vi "Create a constant from terminal.vi"(5 "Terminal Sink":refnum<vi>, 8 "error in (no error)":errorcluster, 10 "Value":variant, 11 "Constant from this terminal":refnum<vi>) -> (0 "error out":errorcluster, 2 "Terminal":refnum<vi>, 3 "Const Refnum":refnum<vi>)   [LabVIEW 2014, in "Scripting Tools.lvlib"]
doc: "Create a constant based on the type of <b>Constant from this terminal</b>. If <b>Value</b> is wired with the same type as the terminal, then the constant has the name and value of this data rather than the name and value associated with the terminal."
uses:
  <userlib>/_LAVACR/Scripting Tools/Scripting Tools.lvlib
  <vilib>/Utility/VariantDataType/VariantType.lvlib
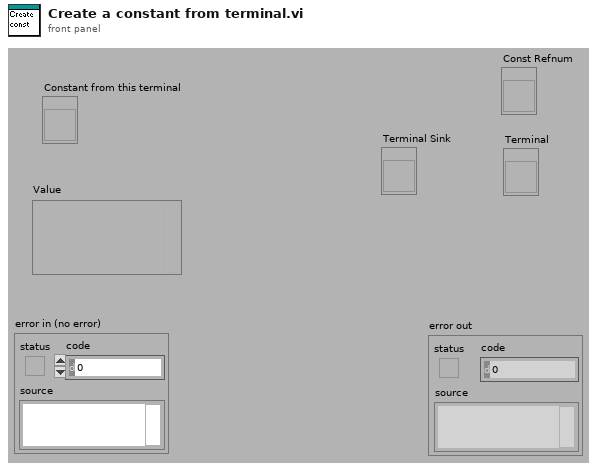
[diagram p1: front panel]
types:
  T1 = typedef "VariantType.lvlib/Type.ctl" = enum8{"Invalid Type", "Void", "I8", "I16", "I32", "I64", "U8", "U16", "U32", "U64", "Single Float", "Double Float", "Extended Float", "Single Complex", "Double Complex", "Extended Complex", "Enum U8", "Enum U16", "Enum U32", "Enum U64", "Single Float With Unit", "Double Float With Unit", "Extended Float With Unit", "Single Complex with Unit", "Double Complex with Unit", "Extended Complex with Unit", "Boolean", "String", "Path", "Picture", "Tag", "Array", "Cluster", "Variant", "LV Variant", "Waveform", "Timestamp", "Digital Waveform", "Digital Data", "ExpressData", "Refnum", "External Data", "VI", "Poly VI", "LabVIEW Class Instance", "Fixed Point"}
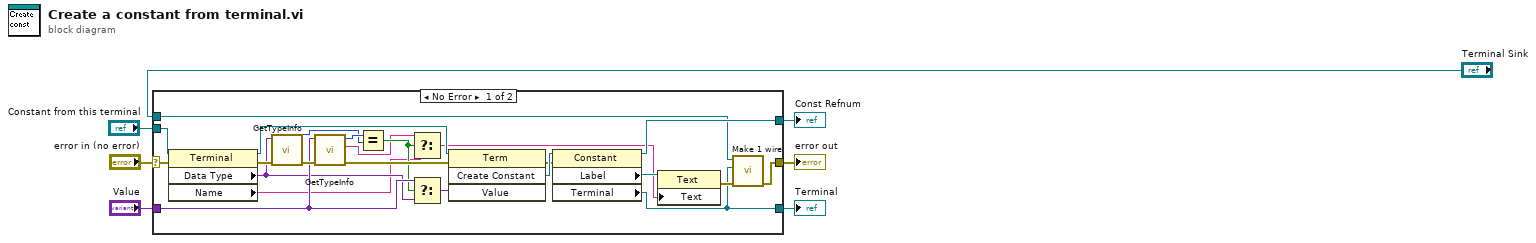
[diagram p0: block diagram]
diagram:
  n1 = case shown="No Error" "error in (no error)" {
    selector: "error in (no error)" -> [w18 w31]
    tunnel: [w29 w31] -> w6
    tunnel: [w27 _] -> w4
    tunnel: [w30 _] -> w5
    tunnel: "Terminal Sink" -> [w26 _]
    tunnel: "Constant from this terminal" -> [w19 _]
    tunnel: "Value" -> [w15 _]
    frame No Error {
      n2 = property class="Terminal"(reference=w19, error in=w18) -> (reference out=w20:refnum<vi>, error out=w22:errorcluster, "Data Type"=w14:variant, "Name"=w9:string)
      n3 = call <vilib>:"GetTypeInfo.vi"("error in (no error)"=w22, "Variant"=w14) -> ("error out"=w21:errorcluster, "Type Enum"=w16:T1)  [unwired: 8 out]
      n4 = call <vilib>:"GetTypeInfo.vi"("error in (no error)"=w21, "Variant"=w15) -> ("error out"=w12:errorcluster, "Name"=w10:string, "Type Enum"=w17:T1)  [unwired: 7 out]
      n5 = Equal?(x=w17, y=w16) -> (x = y?=w11:bool)
      n6 = Select(t=w10, s=w11, f=w9) -> (s? t:f=w8:string)
      n7 = Select(t=w15, s=w11, f=w14) -> (s? t:f=w13:variant)
      n8 = invoke class="Term" method="Create Constant"(reference=w20, error in=w12, "Value"=w13) -> (error out=w23:errorcluster, "Create Constant"=w24:refnum<vi>)  [unwired: 1 in, 2 out]
      n9 = property class="Constant"(reference=w24, error in=w23) -> (reference out=w30:refnum<vi>, "Label"=w25:refnum<vi>, "Terminal"=w27:refnum<vi>)  [unwired: 1 out]
      n10 = property class="Text"(reference=w25, "Text"=w8) -> (error out=w28:errorcluster)  [unwired: 1 in, 1 out]
      n11 = call <userlib>:"Make 1 wire.vi"("error in"=w28, "Wire Terminal 2"=w27, "Wire Terminal 1"=w26) -> ("error out"=w29:errorcluster)  [unwired: 8 out]
    }
    frame Error {
    }
  }
  "error out" <- w6
  "Const Refnum" <- w5
  "Terminal" <- w4
